vi "标定数据保存.vi"(10 "Section":string="传感器对中台", 11 "枚举":enum16{"读取", "保存"}(ring)) -> ()   [LabVIEW 2020]
uses:
  Global_Variable/Global.vi
panel:
  in  "工位二扭矩偏移":cluster{"正向":dbl, "逆向":dbl}
  in  "工位一扭矩偏移":cluster{"正向":dbl, "逆向":dbl}
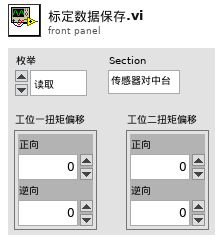
[diagram p1: front panel]
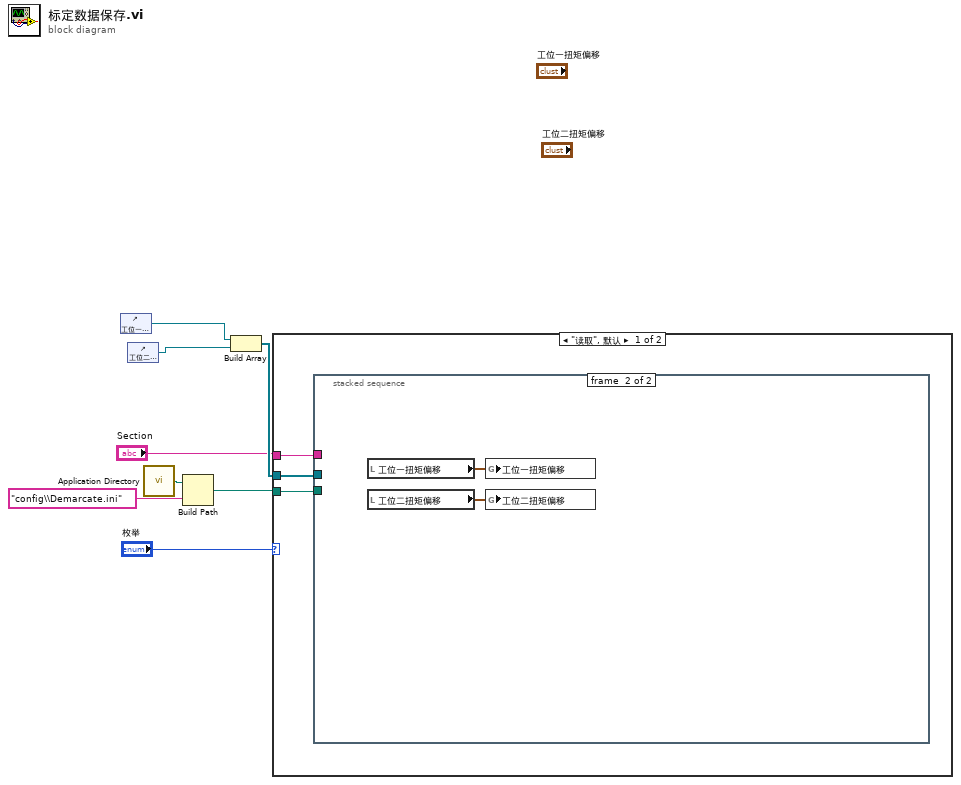
[diagram p0: block diagram]
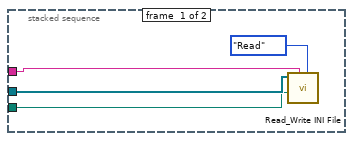
[diagram p2: hidden frame]
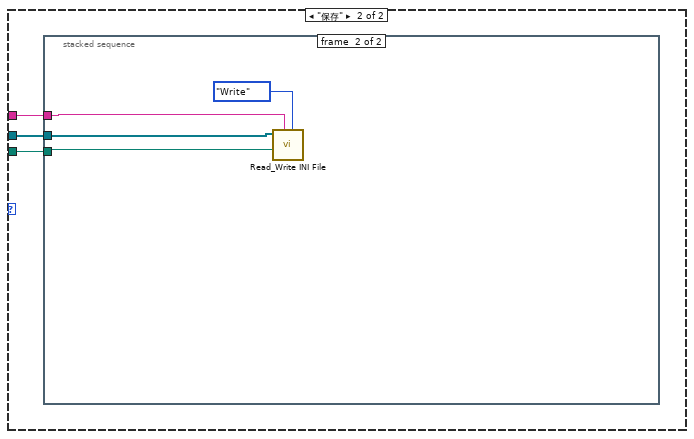
[diagram p3: hidden frame]
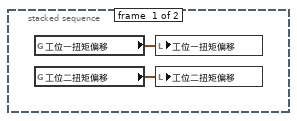
[diagram p4: hidden frame]
diagram:
  n1 = control-ref of="工位一扭矩偏移"() -> (w6:refnum<vi>)
  n2 = control-ref of="工位二扭矩偏移"() -> (w7:refnum<vi>)
  n3 = call <vilib>:"Application Directory.vi"() -> ("Application Directory"=w4:path)
  n4 = Build Path(base path=w4, name or relative path="config\\Demarcate.ini" ("名称或相对路径")) -> (appended path=w2:path)
  n5 = Build Array(w6, w7) -> (w5:refnum<vi>[])
  n6 = case shown="\"读取\", 默认" "枚举" {
    tunnel: w5 -> [w10 w20]
    tunnel: w2 -> [w9 w19]
    tunnel: "Section" -> [w11 w18]
    frame "读取", Default {
      n7 = stacked-sequence {
        tunnel: w10 -> [w14 _]
        tunnel: w9 -> [w13 _]
        tunnel: w11 -> [w15 _]
        frame #0 {
          n8 = call "Read_Write INI File.vi"("Mode"=enum16{"Read", "Write"}."Read", "Section"=w15, "Filepath"=w13, "Ctl Refnum"=w14) -> ()  [unwired: 7 in, 1 out]
        }
        frame #1 {
          n9 = local read "工位一扭矩偏移"() -> (w17:cluster{"正向":dbl, "逆向":dbl})
          n10 = local read "工位二扭矩偏移"() -> (w16:cluster{"正向":dbl, "逆向":dbl})
          n11 = global write "Global.vi" "工位一扭矩偏移"(w17) -> ()
          n12 = global write "Global.vi" "工位二扭矩偏移"(w16) -> ()
        }
      }
    }
    frame "保存" {
      n13 = stacked-sequence {
        tunnel: w20 -> [_ w24]
        tunnel: w19 -> [_ w23]
        tunnel: w18 -> [_ w26]
        frame #0 {
          n14 = global read "Global.vi" "工位一扭矩偏移"() -> (w22:cluster{"正向":dbl, "逆向":dbl})
          n15 = global read "Global.vi" "工位二扭矩偏移"() -> (w21:cluster{"正向":dbl, "逆向":dbl})
          n16 = local write "工位一扭矩偏移"(w22) -> ()
          n17 = local write "工位二扭矩偏移"(w21) -> ()
        }
        frame #1 {
          n18 = call "Read_Write INI File.vi"("Mode"=enum16{"Read", "Write"}."Write", "Section"=w26, "Filepath"=w23, "Ctl Refnum"=w24) -> ()  [unwired: 7 in, 1 out]
        }
      }
    }
  }
